vi "TimerCaseFunctionnal.vi"() -> ()   [LabVIEW 2023]
panel:
  out "Present":dbl
  out "Time elapsed in current phase [s]":dbl
  in  "Start Process":bool
  in  "Time Adsorption [Min]":dbl
  out "Adsorption":bool
  out "Heating":bool
  out "Desorption":bool
  out "Cooling":bool
  out "Idle":bool
  in  "Stop process":bool
  in  "stop 4":bool
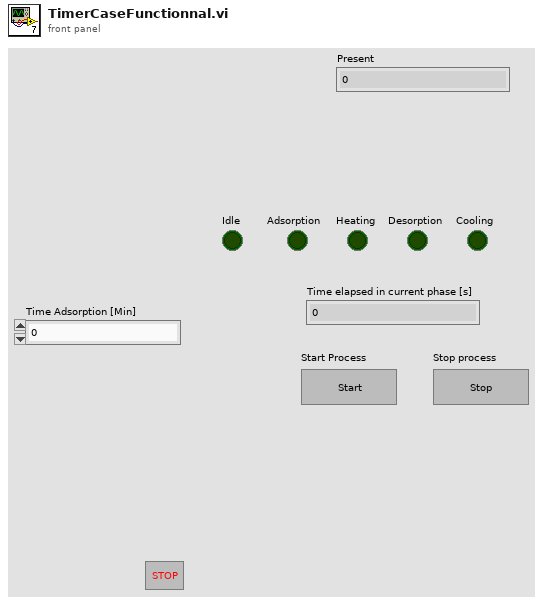
[diagram p1: front panel]
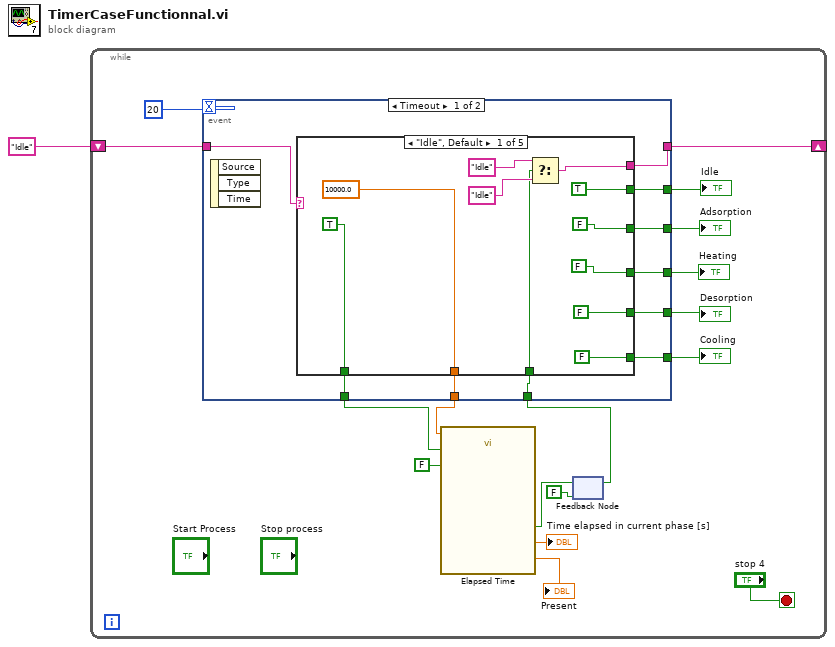
[diagram p0: block diagram]
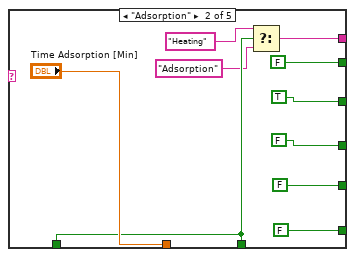
[diagram p2: hidden frame]
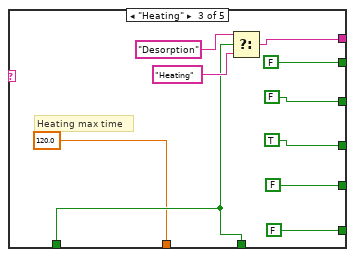
[diagram p3: hidden frame]
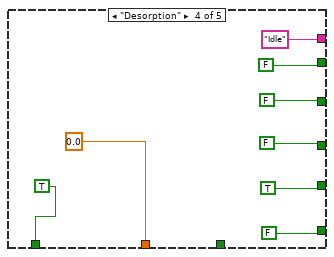
[diagram p4: hidden frame]
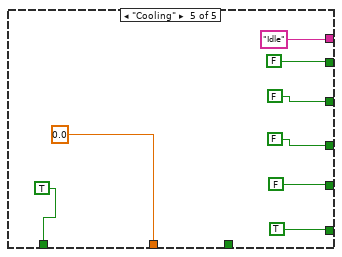
[diagram p5: hidden frame]
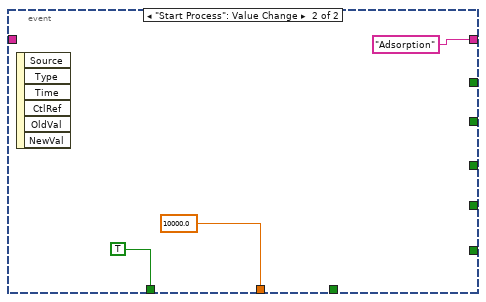
[diagram p6: hidden frame]
diagram:
  n1 = while {
    shift-right: [w10] -> _
    shift-left: "Idle" ("f") -> [w9]
    stop <- "stop 4" stop-if-true
    n2 = feedback #1(FALSE) -> (w5:bool)
    n3 = event shown="[0] Timeout" {
      selector: _ -> [_ _]
      dyn-events: _ -> [_ _]
      timeout: 20 -> [_ _]
      tunnel: [w28 _] -> w18
      tunnel: [w27 _] -> w17
      tunnel: [w26 _] -> w16
      tunnel: [w25 _] -> w15
      tunnel: [w24 _] -> w14
      tunnel: [w23 10000.0] -> w13
      tunnel: [w22 TRUE] -> w12
      tunnel: w5 -> [w21 _]
      tunnel: [w19 "Adsorption" ("f")] -> w10
      tunnel: w9 -> [w20 _]
      event Timeout {
        n4 = event-data() -> ()  [unwired: 1 in, 3 out]
        n5 = case shown="\"Idle\", Default" w20 {
          tunnel: [w32 w44 w52 "Idle" "Idle"] -> w19
          tunnel: [TRUE FALSE FALSE FALSE FALSE] -> w28
          tunnel: [FALSE TRUE FALSE FALSE FALSE] -> w27
          tunnel: [FALSE FALSE TRUE FALSE FALSE] -> w26
          tunnel: [FALSE FALSE FALSE TRUE FALSE] -> w25
          tunnel: [FALSE FALSE FALSE FALSE TRUE] -> w24
          tunnel: [10000.0 "Time Adsorption [Min]" 120.0 0.0 0.0] -> w23
          tunnel: [TRUE w41 w51 TRUE TRUE] -> w22
          tunnel: w21 -> [w29 w41 w51 _ _]
          frame "Idle", Default {
            n6 = Select(t="Idle", s=w29, f="Idle") -> (s? t:f=w32:string)
          }
          frame "Adsorption" {
            n7 = Select(t="Heating", s=w41, f="Adsorption") -> (s? t:f=w44:string)
          }
          frame "Heating" {
            # "Heating max time"
            n8 = Select(t="Desorption", s=w51, f="Heating") -> (s? t:f=w52:string)
          }
          frame "Desorption" {
          }
          frame "Cooling" {
          }
        }
      }
      event "Start Process": Value Change {
        n9 = event-data() -> ()  [unwired: 1 in, 6 out]
      }
    }
    "Adsorption" <- w17
    "Heating" <- w16
    "Desorption" <- w15
    "Cooling" <- w14
    "Idle" <- w18
    n10 = call "Elapsed Time"("Time Target (s)"=w13, "Reset"=w12, "Auto Reset"=FALSE) -> ("Present (s)"=→"Present":dbl, "Elapsed Time (s)"=→"Time elapsed in current phase [s]":dbl, "Time has Elapsed"=w6:bool)  [unwired: 9 in, 5 out]
    n11 = feedback-in #1(w6) -> ()
  }
